vi "Build and Install in LabVIEW.vi"() -> ()   [LabVIEW 2013]
uses:
  <vilib>/JKI/VIPM API/VIPM API_vipm_api.lvlib
panel:
  in  "Build":bool
  in  "LabVIEW Version (to Install into)":string(combo)="13.0"
  out "error out":errorcluster
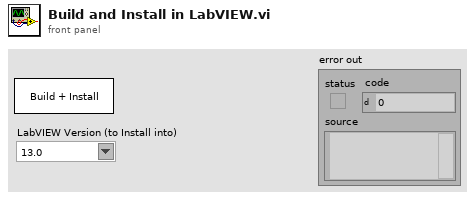
[diagram p1: front panel]
types:
  T1 = typedef "VIPM API_vipm_api.lvlib/LabVIEW Target Info Cluster_vipm_api.ctl" = cluster{"Version":string, "Connection Tested":bool, "Disabled":bool}
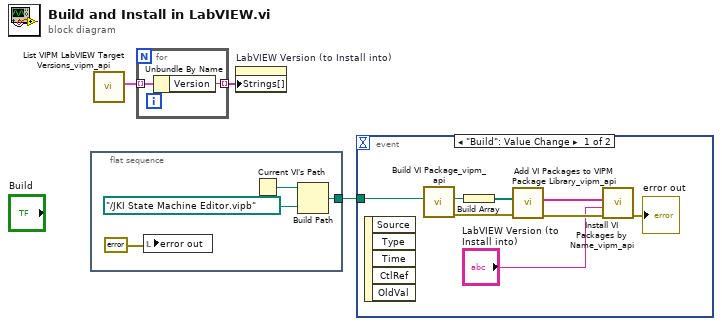
[diagram p0: block diagram]
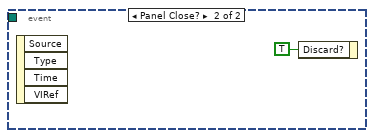
[diagram p2: hidden frame]
diagram:
  n1 = flat-sequence {
    tunnel: [w5] -> w3
    frame #0 {
      n2 = local write "error out"(errorcluster {"status"=FALSE, "code"=0, "source"=""} ("error out")) -> ()
      n3 = Current VI's Path() -> (path=w7:path)
      n4 = Build Path(base path=w7, name or relative path=path "../JKI State Machine Editor.vipb" ("path")) -> (appended path=w5:path)
    }
  }
  n5 = call <vilib>:"List VIPM LabVIEW Target Versions_vipm_api.vi"() -> ("LabVIEW Target Info"=w2:T1[])  [unwired: 10 in, 1 out]
  n6 = for {
    tunnel: w2 -> [w9] mode=indexing
    tunnel: [w8] -> w1 mode=indexing
    n7 = Unbundle By Name(w9) -> ("Version"=w8:string)
  }
  n8 = property on="LabVIEW Version (to Install into)" class="CmbBox"("Strings[]"=w1) -> ()  [unwired: 2 in, 2 out]
  n9 = event shown="[0] \"Build\": Value Change" {
    selector: _ -> [_ _]
    dyn-events: _ -> [_ _]
    timeout: _ -> [_ _]
    tunnel: w3 -> [w10 _]
    event "Build": Value Change {
      n10 = event-data() -> ()  [unwired: 1 in, 5 out]
      n11 = call <vilib>:"Build VI Package_vipm_api.vi"("Path to VIPB File"=w10) -> ("error out"=w17:errorcluster, "Build Output"=w16:path)  [unwired: 9 in]
      n12 = Build Array(w16) -> (w15:path[])
      n13 = call <vilib>:"Add VI Packages to VIPM Package Library_vipm_api.vi"("error in (no error)"=w17, "Packages to add to VIPM Library (vipc,vip,ogp)"=w15) -> ("error out"=w14:errorcluster, "Package Names Added"=w13:string[])  [unwired: 8 in]
      n14 = call <vilib>:"Install VI Packages by Name_vipm_api.vi"("error in (no error)"=w14, "LabVIEW Version"="LabVIEW Version (to Install into)", "Package Names to Install []"=w13) -> ("error out"=→"error out":errorcluster)  [unwired: 8 in]
    }
    event Panel Close? {
      n15 = event-data() -> ()  [unwired: 1 in, 4 out]
      n16 = event-data("Discard?"=TRUE) -> ()  [unwired: 1 in, 1 out]
    }
  }
